vi "Run Headless.vi"(8 "error in (no error)":errorcluster, 10 "Mediator Type":refnum<class "IMediator.lvclass">, 11 "RootModel in":refnum<class "RootModel.lvclass">) -> (0 "error out":errorcluster, 3 "RootModel out":refnum<class "RootModel.lvclass">)   [LabVIEW 2020, in "MVA Framework.lvlib" / "RootModel.lvlib" / "RootModel.lvclass"]
doc: "运行无头"
uses:
  RootModel.lvclass
  C:/Program Files/National Instruments/LabVIEW 2020/vi.lib/ActorFramework/Actor/Actor.lvclass
  IMediator/IMediator/IMediator.lvclass
  IObserver/IObserver/IObserver.lvclass/IObserver.ctl
  IModel/IModel/IModel.lvclass/IModel.ctl
  IModel/IModel/IModel.lvclass
  <vilib>/ActorFramework/Actor/Actor.lvclass
  IObserver/IObserver/IObserver.lvclass
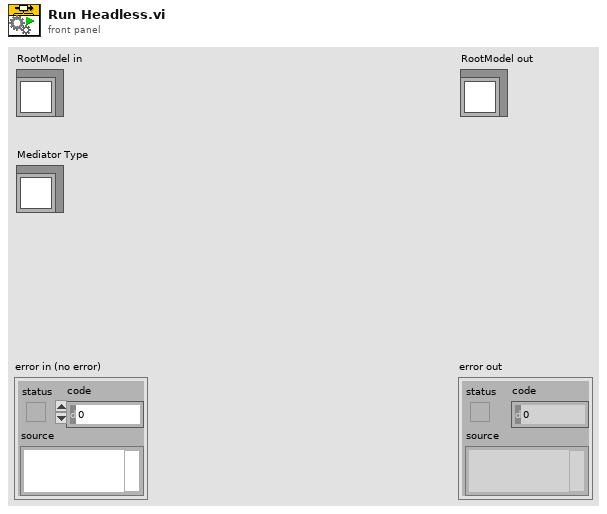
[diagram p1: front panel]
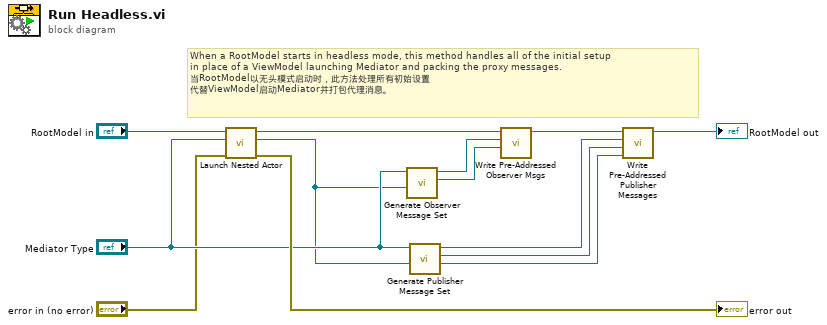
[diagram p0: block diagram]
diagram:
  # "When a RootModel starts in headless mode, this method handles all of the initial setup\nin place of a ViewModel launching Mediator and packing the proxy messages.\n当RootModel以无头模式启动时，此方法处理所有初始设置\n代替ViewModel启动Mediator并打包代理消息。"
  n1 = call <vilib>:"Launch Nested Actor.vi"("error in (no error)"="error in (no error)", "Nested Actor"="Mediator Type", "Caller Actor in"="RootModel in") -> ("error out"=→"error out":errorcluster, "Nested Actor's Enqueuer"=w1:refnum<class "Message Enqueuer.lvclass">, "Caller Actor out"=w12:refnum<class "RootModel.lvclass">)  [unwired: 6 in]
  n2 = call-dynamic "Generate Observer Message Set.vi"("Mediator Enqueuer"=w1, "Mediator Type"="Mediator Type") -> ("Unsubscribe Msg"=w8:refnum<class "Unsubscribe Msg.lvclass">, "Subscribe Msg"=w9:refnum<class "Subscribe Msg.lvclass">)  [unwired: 8 in]
  n3 = call-dynamic "Generate Publisher Message Set.vi"("Mediator Enqueuer"=w1, "IMediator in"="Mediator Type") -> ("Unlock Publication Msg"=w5:refnum<class "Unlock Publication Msg.lvclass">, "Lock Publication Msg"=w4:refnum<class "Lock Publication Msg.lvclass">, "Publish Msg"=w6:refnum<class "Publish Msg.lvclass">)  [unwired: 7 in]
  n4 = call "Write Pre-Addressed Observer Msgs.vi"("Pre-Addressed Unsubscribe Msg"=w8, "Pre-Addressed Subscribe Msg"=w9, "IObserver In"=w12) -> ("IObserver Out"=w11:refnum<class "RootModel.lvclass">)  [unwired: 8 in]
  n5 = call "Write Pre-Addressed Publisher Messages.vi"("Pre-Addressed Unlock Publication Msg"=w5, "Pre-Addressed Lock Publication Msg"=w4, "Pre-Addressed Publish Msg"=w6, "IModel in"=w11) -> ("IModel out"=→"RootModel out":refnum<class "RootModel.lvclass">)  [unwired: 7 in]
